vi "Write Observables to check.vi"(8 "error in (no error)":errorcluster, 10 "Obsv to check":T1(array[cluster]), 11 "Run Instance in":refnum<class "Run Instance.lvclass">) -> (0 "error out":errorcluster, 3 "Run Instance out":refnum<class "Run Instance.lvclass">)   [LabVIEW 2020, in "CIRCUS_uServices.lvlib" / "Run Utilities.lvlib" / "Run Instance.lvclass"]
uses:
  Run Instance.lvclass
  Run Instance.lvclass/Run Instance.ctl
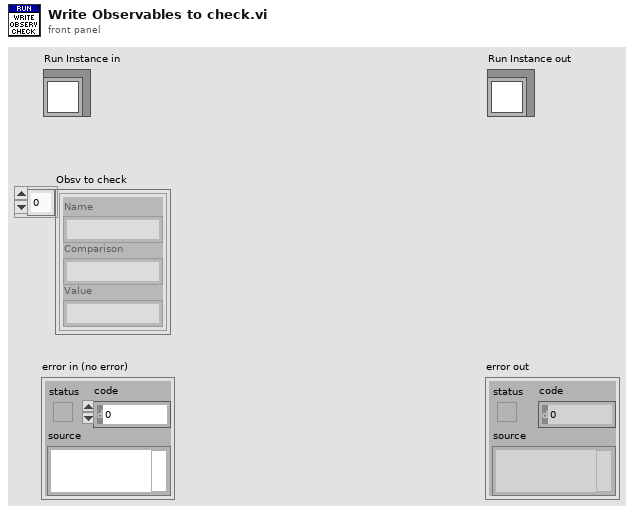
[diagram p1: front panel]
types:
  T1 = cluster{"Name":string, "Comparison":string, "Value":string}[]
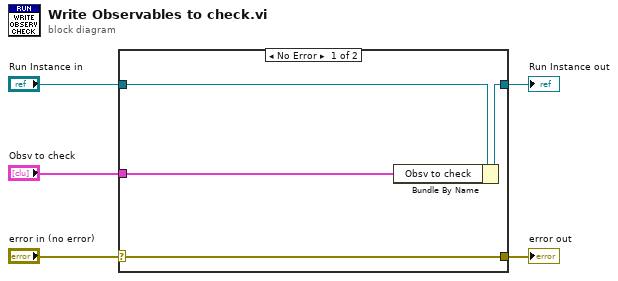
[diagram p0: block diagram]
diagram:
  n1 = case shown="No Error" "error in (no error)" {
    selector: "error in (no error)" -> [w9 w10]
    tunnel: [w9 w10] -> w4
    tunnel: [w7 w11] -> w2
    tunnel: "Run Instance in" -> [w8 w11]
    tunnel: "Obsv to check" -> [w6 _]
    frame No Error {
      n2 = Bundle By Name(cluster=w8, "Obsv to check"=w6) -> (w7:refnum<class "Run Instance.lvclass">)
    }
    frame Error {
    }
  }
  "error out" <- w4
  "Run Instance out" <- w2
